vi "Initialize Front Panel.vi"(8 "error in (no error)":errorcluster, 11 "LeftListboxViewManager in":refnum<class "LeftListboxViewManager.lvclass">) -> (0 "error out":errorcluster, 3 "LeftListboxViewManager out":refnum<class "LeftListboxViewManager.lvclass">)   [LabVIEW 2015, in "LeftListboxViewManager.lvlib" / "LeftListboxViewManager.lvclass"]
doc: "<License>\nCopyright © 2017 Composed Systems, LLC | All rights reserved\nwww.composed.io\n\nAuthor: Ethan Stern <ethan.stern@composed.io>\n\nThis software is provided \"AS IS\" WITHOUT WARRANTIES, either express or implied, AND IS FOR EDUCATIONAL PURPOSES ONLY.\n</License>"
uses:
  LeftListboxViewManager.lvclass
  Framework/IViewManager/IViewManager/IViewManager.lvclass/IViewManager.ctl
  LeftListboxViewManager.lvclass/LeftListboxViewManager.ctl
  Framework/IViewable/IViewable Messages/Insert Front Panel Msg/Insert Front Panel Msg.lvclass/Insert Front Panel Msg.ctl
  <vilib>/ActorFramework/Message Enqueuer/Message Enqueuer.lvclass/Message Enqueuer.ctl
  <vilib>/ActorFramework/Message Enqueuer/Enqueue.vi
  <vilib>/ActorFramework/Message Priority Queue/Priority Enqueue.vi
  Framework/IViewManager/IViewManager/IViewManager.lvclass
  Framework/IViewable/IViewable Messages/Insert Front Panel Msg/Insert Front Panel Msg.lvclass
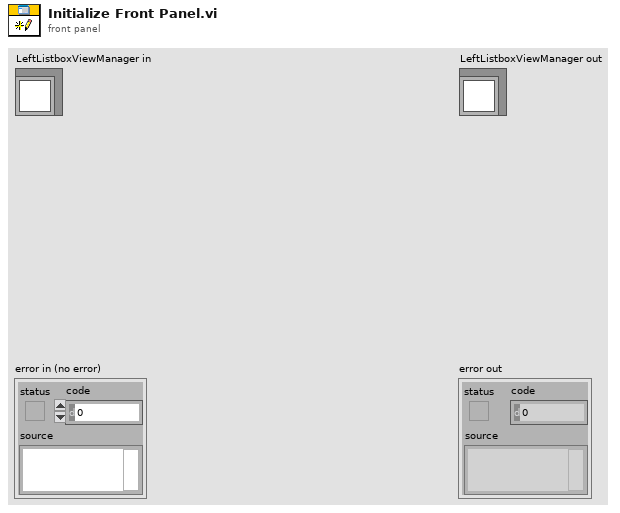
[diagram p1: front panel]
types:
  T1 = typedef "IViewable.lvlib/ProtectedSubpanel.lvclass/Protected Subpanel Reference.ctl" = refnum<data-value>
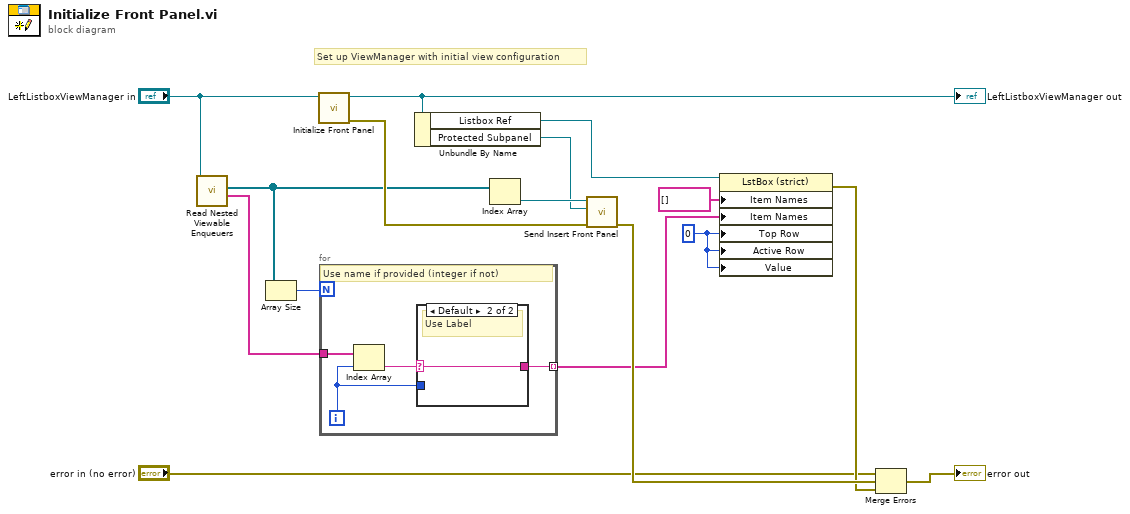
[diagram p0: block diagram]
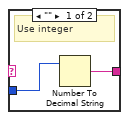
[diagram p2: hidden frame]
diagram:
  w10 = 0 ("Top Row")
  # "Set up ViewManager with initial view configuration"
  n1 = call "Read Nested Viewable Enqueuers.vi"("IViewManager in"="LeftListboxViewManager in") -> ("Viewable Names"=w3:string[], "Nested Viewable Enqueuers"=w2:refnum<class "Message Enqueuer.lvclass">[])  [unwired: 9 in]
  n2 = Array Size(array=w2) -> (size(s)=w1:i32)
  n3 = call-parent "Initialize Front Panel.vi"("IViewable in"="LeftListboxViewManager in") -> ("error out"=w8:errorcluster, "IViewable out"=w7:refnum<class "LeftListboxViewManager.lvclass">)  [unwired: 9 in]
  "LeftListboxViewManager out" <- w7
  n4 = for {
    N: w1 -> [_]
    tunnel: [w20] -> w9 mode=indexing
    tunnel: w3 -> [w17]
    i -> [w19]
    # "Use name if provided (integer if not)"
    n5 = Index Array(array=w17, index=w19) -> (element=w18:string)
    n6 = case shown="Default" w18 {
      selector: w18 -> [_ w23]
      tunnel: [w21 w23] -> w20
      tunnel: w19 -> [w22 _]
      frame "" {
        # "Use integer"
        n7 = Number To Decimal String(number=w22) -> (decimal integer string=w21:string)  [unwired: 1 in]
      }
      frame Default {
        # "Use Label"
      }
    }
  }
  n8 = Unbundle By Name(w7) -> ("Listbox Ref"=w14:refnum<vi>, "Protected Subpanel"=w15:T1)
  n9 = Index Array(array=w2) -> (element=w16:refnum<class "Message Enqueuer.lvclass">)  [unwired: 1 in]
  n10 = call "Send Insert Front Panel.vi"("error in (no error)"=w8, "Protected Subpanel"=w15, "Message Enqueuer"=w16) -> ("error out"=w12:errorcluster)  [unwired: 7 in, 1 out]
  n11 = property class="LstBox (strict)"(reference=w14, "Item Names"=string[] [], "Item Names"=w9, "Top Row"=w10, "Active Row"=w10, "Value"=w10) -> (error out=w11:errorcluster)  [unwired: 1 in, 1 out]
  n12 = Merge Errors("error in (no error)", w12, w11) -> (→"error out":errorcluster)
